vi "averaged_stokes_acquisition.vi"(0 "Motor \"Name\"":string="1", 2 "VISA resource name":refnum<visa-resource-name>="COM3", 5 "Encoder Pulses per Degree":i32=398, 7 "Number of Angles":i32=8, 9 "Number of Measures":i32=10, 11 "ICImagingControl In":refnum<k7>, 13 "Saving Path":path=path "C:/Users/Usuario/OneDrive - Universitat de Barcelona/PhD") -> ()   [LabVIEW 2024]
panel:
  out "Image":T1(plugin-control)
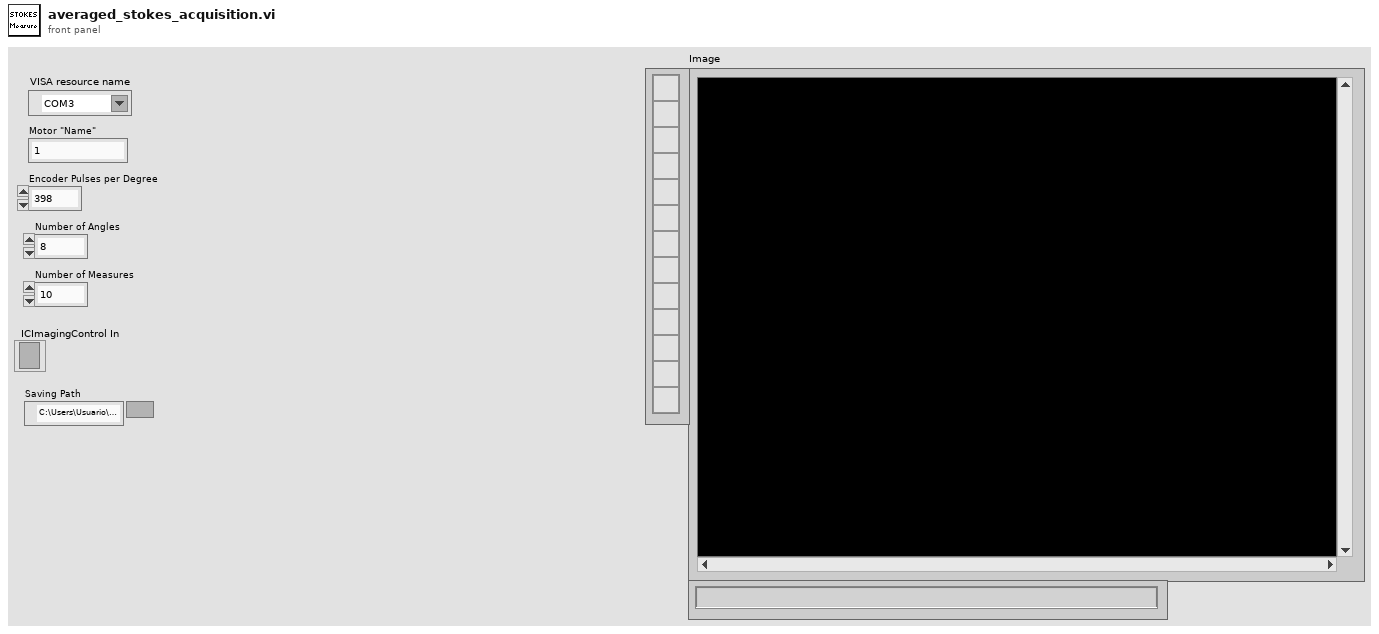
[diagram p1: front panel]
types:
  T1 = typedef "IMAQ Image.ctl" = refnum<image>
  T2 = typedef "Image Type" = u32
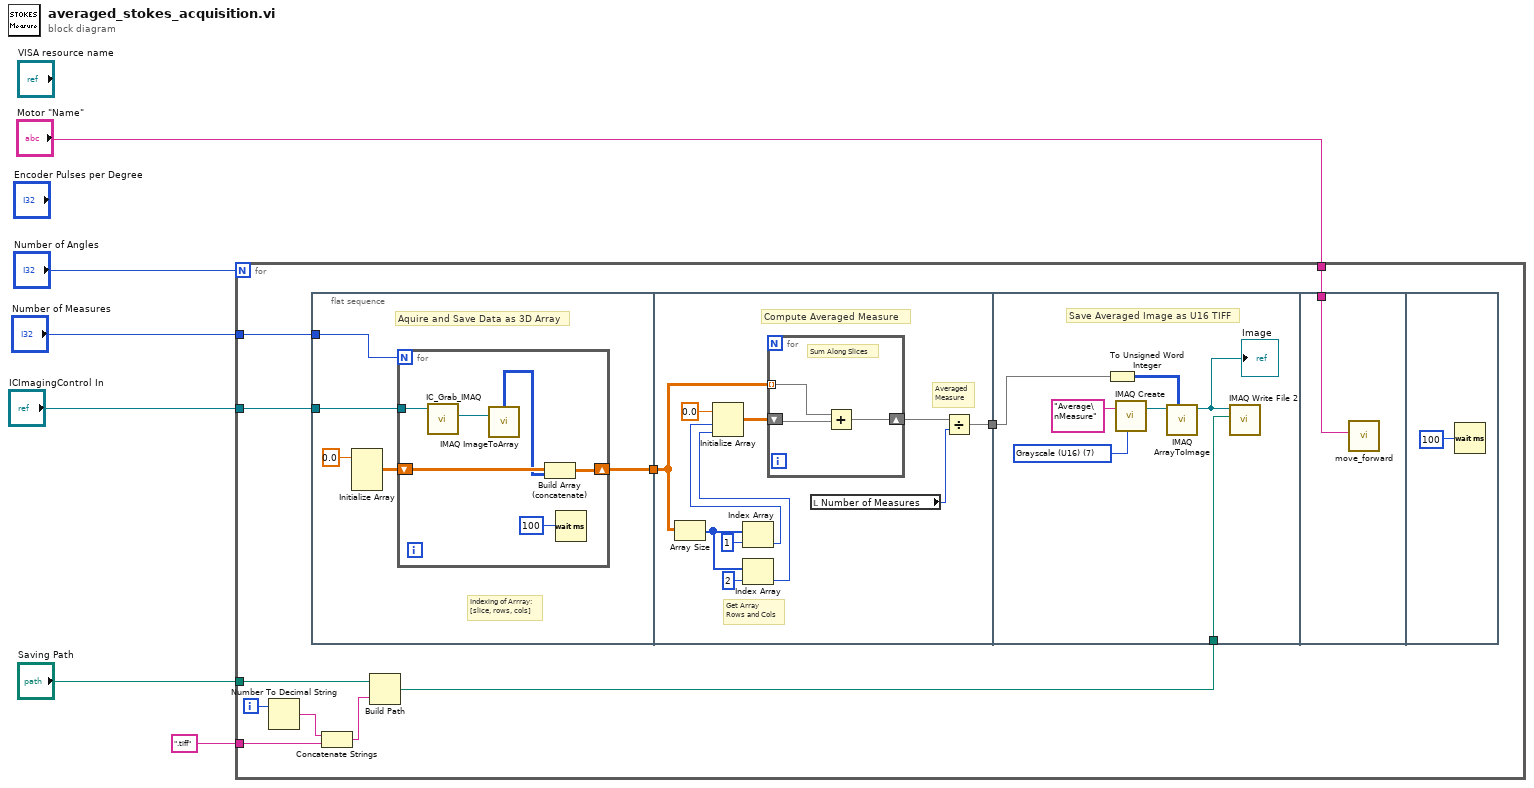
[diagram p0: block diagram]
diagram:
  n1 = for {
    N: "Number of Angles" -> [_]
    tunnel: ".tiff" -> [w14]
    tunnel: "Saving Path" -> [w12]
    tunnel: "ICImagingControl In" -> [w13]
    tunnel: "Number of Measures" -> [w11]
    tunnel: "Motor \"Name\"" -> [w7]
    i -> [w17]
    n2 = Number To Decimal String(number=w17) -> (decimal integer string=w16:string)  [unwired: 1 in]
    n3 = flat-sequence {
      tunnel: w13 -> [w22]
      tunnel: w11 -> [w20]
      tunnel: [w19] -> w10
      tunnel: w10 -> [w33]
      tunnel: [w29] -> w9
      tunnel: w9 -> [w45]
      tunnel: w8 -> [w49]
      tunnel: w7 -> [w50]
      frame #0 {
        # "Aquire and Save Data as 3D Array"
        # "Indexing of Arrray:\n[slice, rows, cols]"
        n4 = Initialize Array(0.0) -> (w21:dbl[][][])  [unwired: 3 in]
        n5 = for {
          N: w20 -> [_]
          tunnel: w22 -> [w26]
          shift-right: [w23] -> w19
          shift-left: w21 -> [w27]
          n6 = call <userlib>:"IC_Grab_IMAQ.vi"("ICImagingControl In"=w26) -> ("Image Out"=w25:T1)  [unwired: 2 in, 3 out]
          n7 = call "IMAQ ImageToArray"("Image"=w25) -> ("Image Pixels (U8)"=w24:u8[][])  [unwired: 3 in, 4 out]
          n8 = Build Array (concatenate)(w27, w24) -> (w23:dbl[][][])
          n9 = Wait (ms)(milliseconds to wait=u32 100) -> ()  [unwired: 1 out]
        }
      }
      frame #1 {
        # "Compute Averaged Measure"
        # "Averaged\nMeasure"
        # "Get Array \nRows and Cols"
        n10 = Array Size(array=w33) -> (size(s)=w38:i32[])
        n11 = Index Array(array=w38, index=1) -> (element=w35:i32)
        n12 = Index Array(array=w38, index=2) -> (element=w34:i32)
        n13 = Initialize Array(0.0 ("element"), w35, w34) -> (w32:dbl[][])
        n14 = for {
          tunnel: w33 -> [w41] mode=indexing
          shift-right: [w40] -> w31
          shift-left: w32 -> [w42]
          # "Sum Along Slices"
          n15 = Add(x=w41, y=w42) -> (x+y=w40:dbl[][])
        }
        n16 = local read "Number of Measures"() -> (w30:i32)
        n17 = Divide(x=w31, y=w30) -> (x/y=w29:dbl[][])
      }
      frame #2 {
        w46 = T2 7 items=["Grayscale (U8)", "Grayscale (I16)", "Grayscale (SGL)", "Complex (CSG)", "RGB (U32)", "HSL (U32)", "RGB (U64)", "Grayscale (U16)"] ("Image Type")
        # "Save Averaged Image as U16 TIFF"
        n18 = To Unsigned Word Integer(number=w45) -> (unsigned 16bit integer=w44:u16[][])
        n19 = call "IMAQ Create"("Image Name"="Average\nMeasure", "Image Type"=w46) -> ("New Image"=w47:T1)  [unwired: 3 in, 1 out]
        n20 = call "IMAQ ArrayToImage"("Image Pixels (U16)"=w44, "Image"=w47) -> ("Image Out"=w43:T1)  [unwired: 8 in, 1 out]
        "Image" <- w43
        n21 = call-poly "IMAQ Write File 2"("File Path"=w49, "Image"=w43) -> ()  [unwired: 8 in, 2 out]
      }
      frame #3 {
        n22 = call "move_forward.vi"("Motor \"Name\""=w50) -> ()  [unwired: 9 in, 2 out]
      }
      frame #4 {
        n23 = Wait (ms)(milliseconds to wait=u32 100) -> ()  [unwired: 1 out]
      }
    }
    n24 = Concatenate Strings(w16, w14) -> (w15:string)
    n25 = Build Path(base path=w12, name or relative path=w15) -> (appended path=w8:path)
  }
